vi "LibXML_AllMatchNodes.vi"(8 "error in":errorcluster, 9 "XPath":string, 10 "root node":u32, 11 "doc":u32) -> (0 "error out":errorcluster, 2 "Matched Nodes":u32[](array[numeric]), 3 "doc out":u32)   [LabVIEW 2019, in "Tools.lvlib"]
doc: "Get all matched nodes to input XPath"
uses:
  Tools.lvlib
  libxml2/LibXML_QueryXPathExpr.vi
  libxml2/LibXML_GetNumberOfNodes.vi
  Error Cluster From Error Code_subroutine.vi
  <vilib>/Utility/error.llb/Trim Whitespace.vi
  LibXML.lvlib
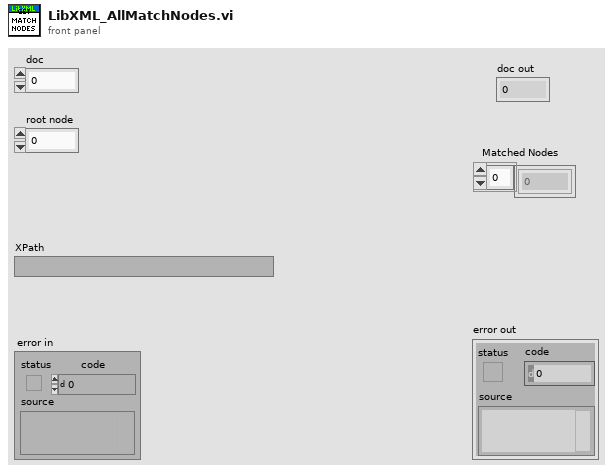
[diagram p1: front panel]
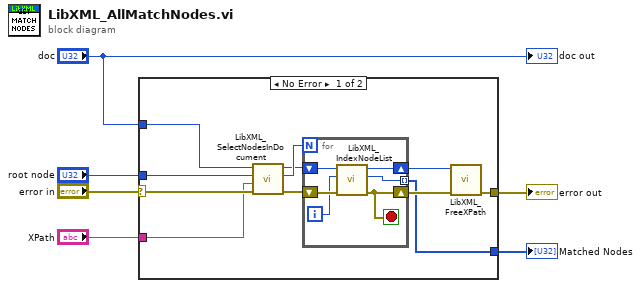
[diagram p0: block diagram]
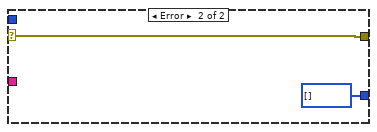
[diagram p2: hidden frame]
diagram:
  n1 = case shown="No Error" "error in" {
    selector: "error in" -> [w10 w25]
    tunnel: [w12 u32[] []] -> w6
    tunnel: [w11 w25] -> w5
    tunnel: "XPath" -> [w9 _]
    tunnel: "doc" -> [w8 _]
    tunnel: "root node" -> [w7 _]
    frame No Error {
      n2 = call "LibXML_SelectNodesInDocument.vi"("error in"=w10, "queryString"=w9, "rootnode (root of doc)"=w7, "doc"=w8) -> ("error out"=w13:errorcluster, "length"=w17:i32, "xmlXPathObj"=w14:u32)  [unwired: 2 in, 3 out]
      n3 = for {
        N: w17 -> [_]
        shift-right: [w19] -> w15
        shift-left: w13 -> [w23]
        shift-right: [w20] -> w16
        shift-left: w14 -> [w21]
        tunnel: [w18] -> w12 mode=indexing
        i -> [w22]
        stop <- w19 stop-if-true
        n4 = call "LibXML_IndexNodeList.vi"("error in"=w23, "index"=w22, "XPathObj"=w21) -> ("error out"=w19:errorcluster, "NodePtr"=w18:u32, "XPathObj out"=w20:u32)  [unwired: 6 in]
      }
      n5 = call "LibXML_FreeXPath.vi"("error in"=w15, "XPathObj"=w16) -> ("error out"=w11:errorcluster)  [unwired: 9 in]
    }
    frame Error {
    }
  }
  "Matched Nodes" <- w6
  "error out" <- w5
  "doc out" <- "doc"
